vi "NavDriveStraight3.vi"(7 "Re-Init":bool, 9 "arguments":string[](array[string]), 10 "SensorInputData":T5, 11 "HMI to Control":T1) -> (2 "HMI to Control Out":T1, 3 "SensorInputDataOut":T5, 4 "Done":bool)   [LabVIEW 2014]
uses:
  Typedefs/SensorInputData.ctl
  Typedefs/HMI_to_Control.ctl
  Typedefs/Arm States.ctl
  Typedefs/ClawStates.ctl
  Typedefs/IntakeWheelSenseOrManual.ctl
  scriptlib/auto_data.vi
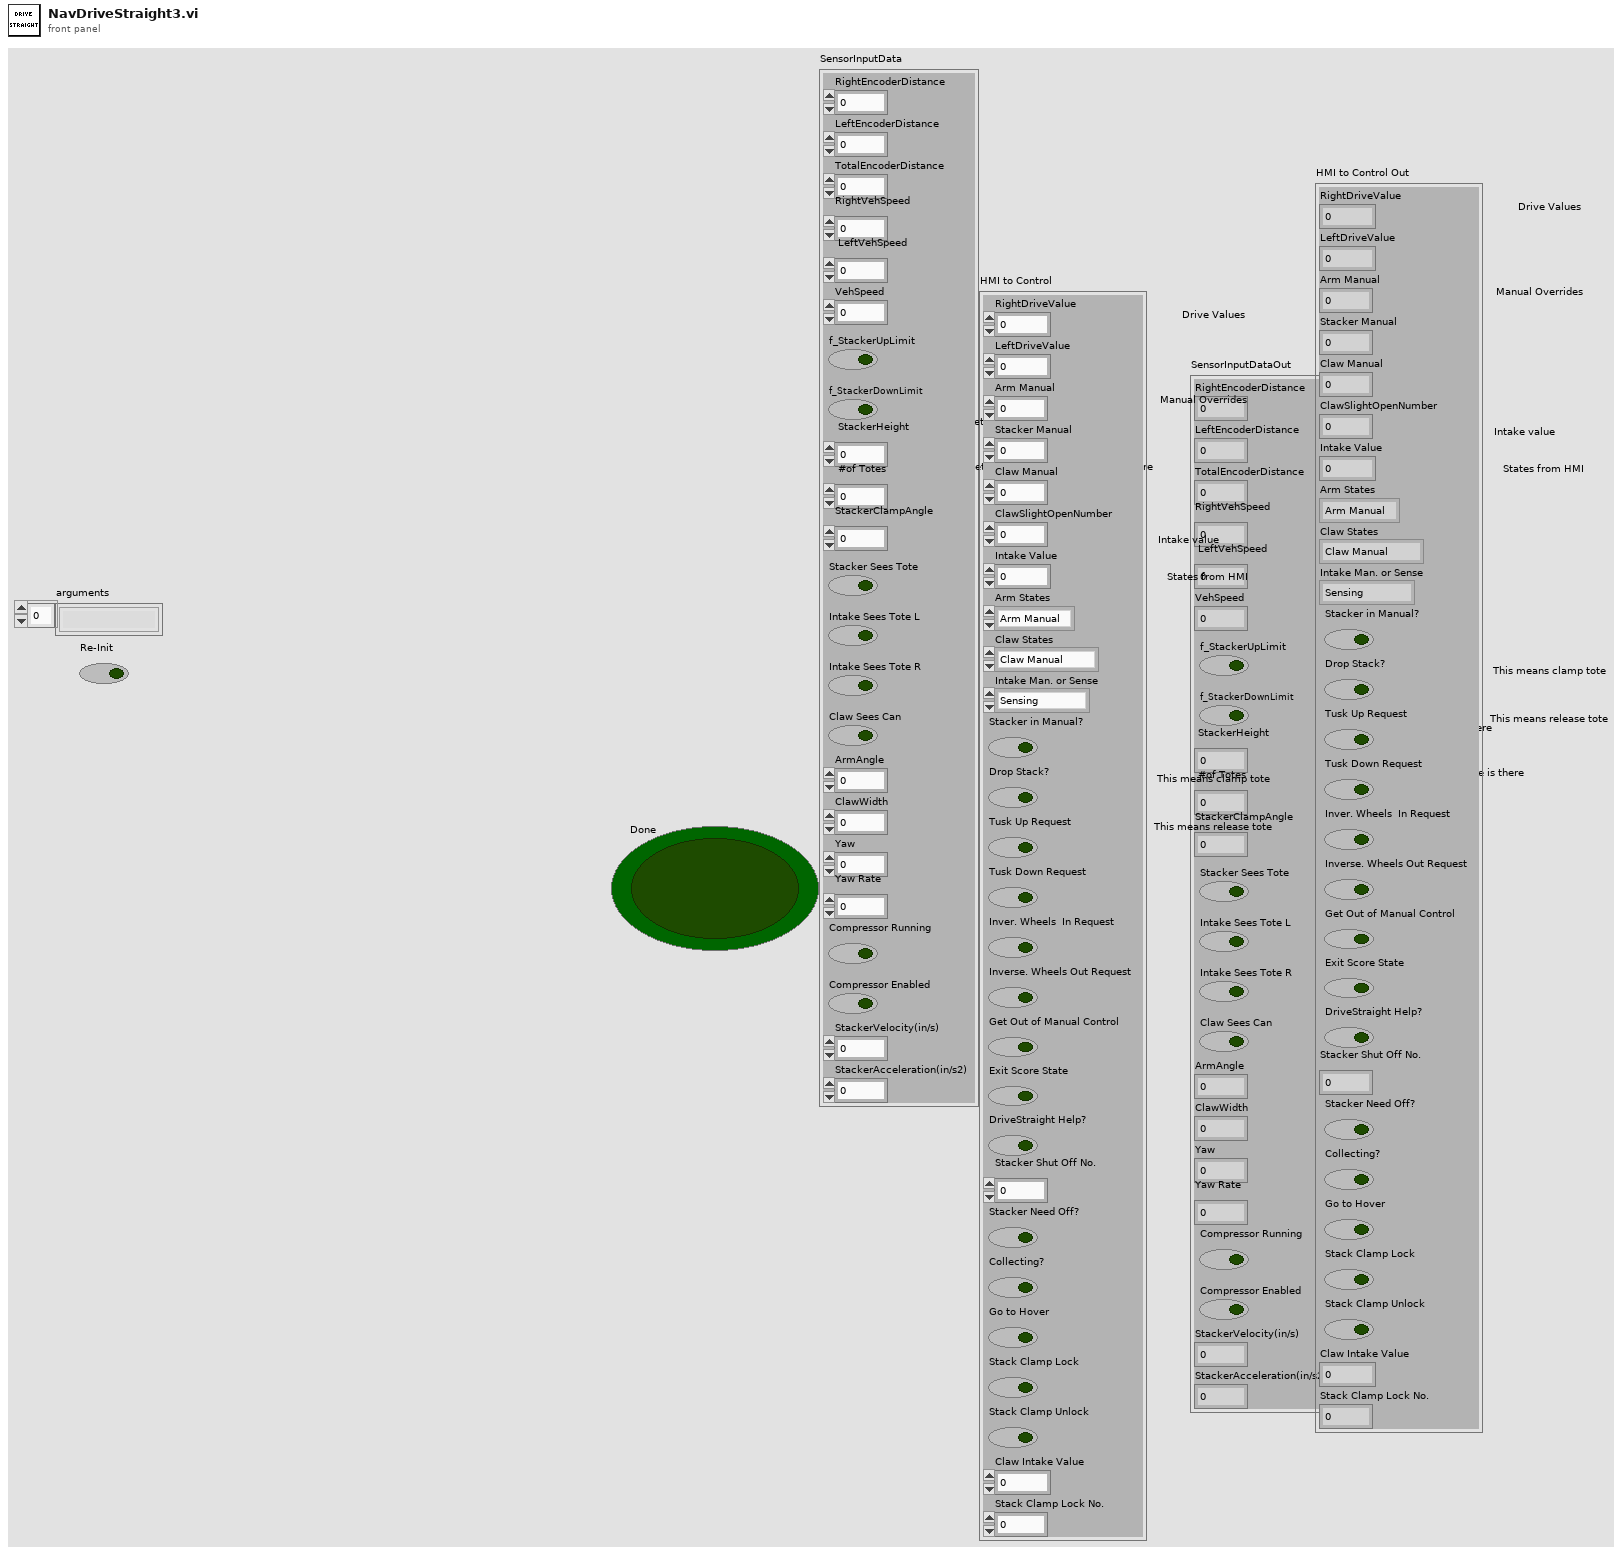
[diagram p1: front panel]
types:
  T1 = typedef "HMI_to_Control.ctl" = cluster{"RightDriveValue":dbl, "LeftDriveValue":dbl, "Arm Manual ":dbl, "Stacker Manual ":dbl, "Claw Manual ":dbl, "ClawSlightOpenNumber":i8, "Intake Value ":i8, "Arm States":T2, "Claw States":T3, "Intake Man. or Sense":T4, "Stacker in Manual?":bool, "Drop Stack? ":bool, "Tusk Up Request":bool, "Tusk Down Request":bool, "Inver. Wheels  In Request":bool, "Inverse. Wheels Out Request ":bool, "Get Out of Manual Control":bool, "Exit Score State":bool, "DriveStraight Help?":bool, "Stacker Shut Off No.":i8, "Stacker Need Off?":bool, "Collecting?":bool, "Go to Hover":bool, "Stack Clamp Lock ":bool, "Stack Clamp Unlock ":bool, "Claw Intake Value ":i8, "Stack Clamp Lock No. ":i8}
  T2 = typedef "Arm States.ctl" = enum16{"Arm Manual ", "Ground", "Step", "1 Tote", "2 Tote", "3 Tote", "4 Tote", "5 Tote", "6 Tote", "Flip Can", "Grab Can in auto"}
  T3 = typedef "ClawStates.ctl" = enum16{"Claw Manual ", "Claw Open", "Claw Closed", "Claw Slight Open", "Tote Get"}
  T4 = typedef "IntakeWheelSenseOrManual.ctl" = enum16{"Sensing", "Manual "}
  T5 = typedef "SensorInputData.ctl" = cluster{"RightEncoderDistance":dbl, "LeftEncoderDistance":dbl, "TotalEncoderDistance":dbl, "RightVehSpeed":dbl, "LeftVehSpeed":dbl, "VehSpeed":dbl, "f_StackerUpLimit":bool, "f_StackerDownLimit":bool, "StackerHeight":dbl, "#of Totes":u8, "StackerClampAngle":dbl, "Stacker Sees Tote":bool, "Intake Sees Tote L":bool, "Intake Sees Tote R":bool, "Claw Sees Can":bool, "ArmAngle":dbl, "ClawWidth":dbl, "Yaw":dbl, "Yaw Rate":dbl, "Compressor Running":bool, "Compressor Enabled":bool, "StackerVelocity(in/s)":dbl, "StackerAcceleration(in/s2)":dbl}
  T6 = cluster{"LeftEncoderDistance":dbl, "RightEncoderDistance":dbl}
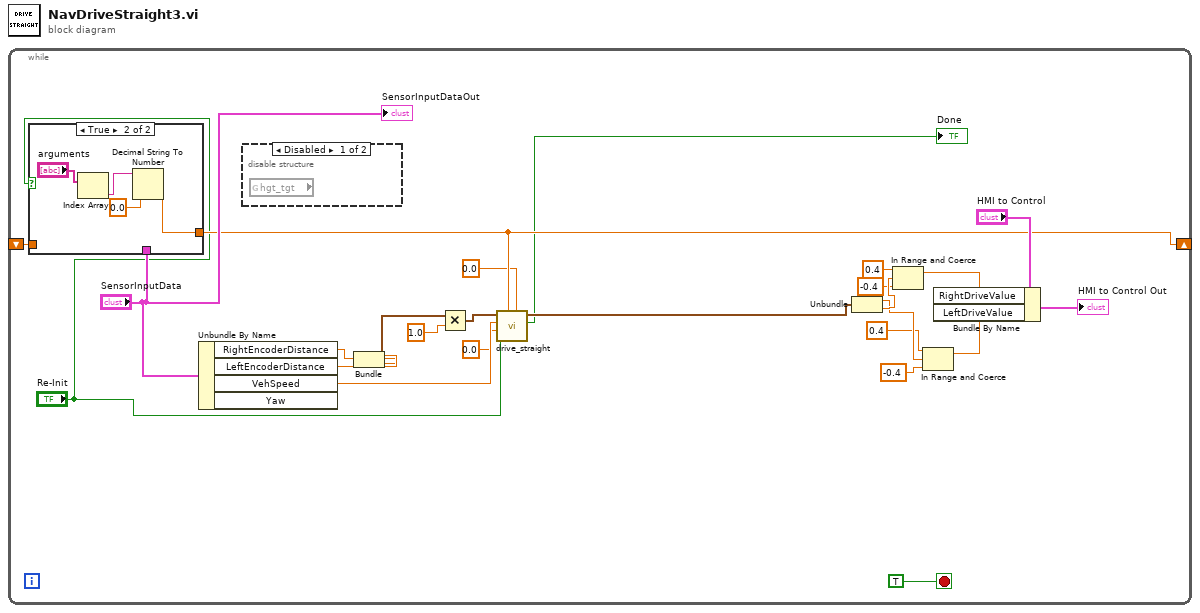
[diagram p0: block diagram]
diagram:
  n1 = while {
    shift-right: [w14] -> _
    shift-left: _ -> [w15]
    stop <- TRUE stop-if-true
    n2 = case shown="True" "Re-Init" {
      tunnel: [w26 w27] -> w14
      tunnel: "SensorInputData" -> [_ _]
      tunnel: w15 -> [w26 _]
      frame False {
      }
      frame True {
        n3 = Index Array(array="arguments") -> (element=w29:string)  [unwired: 1 in]
        n4 = Decimal String To Number(string=w29, default (0L)=0.0) -> (number=w27:dbl)  [unwired: 1 in, 1 out]
      }
    }
    n5 = Unbundle By Name("SensorInputData") -> ("RightEncoderDistance"=w20:dbl, "LeftEncoderDistance"=w21:dbl, "VehSpeed"=w19:dbl)  [unwired: 1 out]
    n6 = disable-structure shown="Disabled" {
      frame Disabled {
        n7 = global read "auto_data.vi" "hgt_tgt"() -> ()  [unwired: 1 out]
      }
      frame Enabled {
      }
    }
    n8 = Bundle("LeftEncoderDistance"=w21, "RightEncoderDistance"=w20) -> (w17:T6)  [unwired: 1 in]
    n9 = Multiply(x=w17, y=1.0) -> (x*y=w18:T6)
    n10 = call "drive_straight.vi"("setpoint_hdg"=0.0, "setpoint_distance"=w14, "reinit"="Re-Init", "gyro_heading"=0.0, "vehspd_avg"=w19, "distances"=w18) -> ("done"=→"Done":bool, "mpower"=w16:cluster{"left":dbl, "right":dbl})  [unwired: 4 in]
    n11 = Unbundle(w16) -> ("left"=w8:dbl, "right"=w12:dbl)
    n12 = In Range and Coerce(upper limit=0.4, x=w12, lower limit=-0.4) -> (coerced(x)=w9:dbl)  [unwired: 1 out]
    n13 = In Range and Coerce(upper limit=0.4, x=w8, lower limit=-0.4) -> (coerced(x)=w5:dbl)  [unwired: 1 out]
    n14 = Bundle By Name(cluster="HMI to Control", "RightDriveValue"=w9, "LeftDriveValue"=w5) -> (→"HMI to Control Out":T1)
    "SensorInputDataOut" <- "SensorInputData"
  }
